vi "Insert Into Subpanel.vi"(8 "error in (no error)":errorcluster, 10 "Active Components":T1, 11 "SubPanel in":refnum<vi>) -> (0 "error out":errorcluster, 2 "VI Reference":refnum<vi>)   [LabVIEW 2020, in "Peek Window.lvlib"]
uses:
  Peek Window.lvlib
  Open Diagram Argument--cluster.ctl
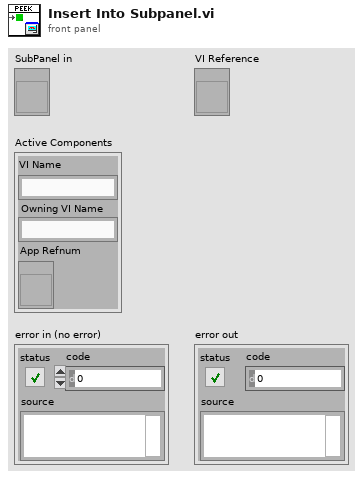
[diagram p1: front panel]
types:
  T1 = typedef "Peek Window.lvlib/Open Diagram Argument--cluster.ctl" = cluster{"VI Name":string, "Owning VI Name":string, "App Refnum":refnum<vi>}
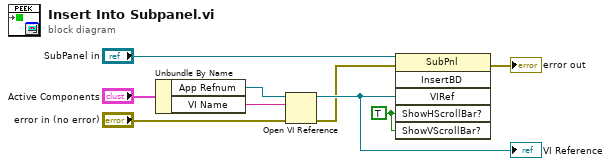
[diagram p0: block diagram]
diagram:
  w6 = TRUE ("ShowHScrollBar")
  n1 = Unbundle By Name("Active Components") -> ("App Refnum"=w2:refnum<vi>, "VI Name"=w1:string)
  n2 = Open VI Reference(application reference (local)=w2, vi path=w1, error in (no error)="error in (no error)") -> (vi reference=w7:refnum<vi>, error out=w5:errorcluster)  [unwired: 3 in]
  "VI Reference" <- w7
  n3 = invoke on="Invoke Node" class="SubPnl" method="InsertBD"(reference="SubPanel in", error in=w5, "VIRef"=w7, "ShowHScrollBar?"=w6, "ShowVScrollBar?"=w6) -> (error out=→"error out":errorcluster)  [unwired: 1 in, 5 out]
